vi "Open Message Handler.vi"(6 "Mouse Position":T1, 7 "User VI Ref":refnum<vi>, 8 "Is Multi-select?":bool, 9 "Remaining Items":refnum<vi>[](array[refnum]), 10 "Affected Items":cluster{"Refnums 1":refnum<vi>[]}, 11 "Menu Refnum":refnum<k9>) -> (3 "Menu Items To Add":T2[](array[typedef]))   [LabVIEW 2020]
doc: "This VI is part of a plug-in for modifying the LabVIEW shortcut menus. This is the builder VI which is called when the shortcut menu is built. It tells LabVIEW which shortcut menu items to add to the menu."
uses:
  <resource>/plugins/PopupMenus/support/Shortcut Menu Item Definition.ctl
  <resource>/plugins/PopupMenus/support/Transaction Control.ctl
  <resource>/plugins/PopupMenus/support/Position In Menu.ctl
  <resource>/plugins/PopupMenus/support/Relative Position.ctl
  <resource>/plugins/PopupMenus/support/Checkmark Status.ctl
  <resource>/plugins/PopupMenus/support/Enabled Menu Item Status.ctl
  <vilib>/Utility/miscctls.llb/LVPositionTypeDef.ctl
panel:
  # "Rules a popup plug-in must follow:\n* This VI's file name must match the file name of the LLB -- only the file extensions should be different.\n* This VI must have debugging disabled or it will be ignored as a plug-in.\n* For all menu items, \"tag suffix + file name of this VI\" must be less than 240 characters.\n* You can disconnect the \"Affected Items\" from the typedef to make the plug-in load faster. The typedef is only there to assist you in keeping this VI and the execution VI using to the same type.\n* All controls on this panel except \"Affected Items\" are locked to prevent accidental edits. Do not change the types or the names of controls other than the elements inside the \"Affected Items\" cluster.\n* See Context Help for more information on the individual controls."
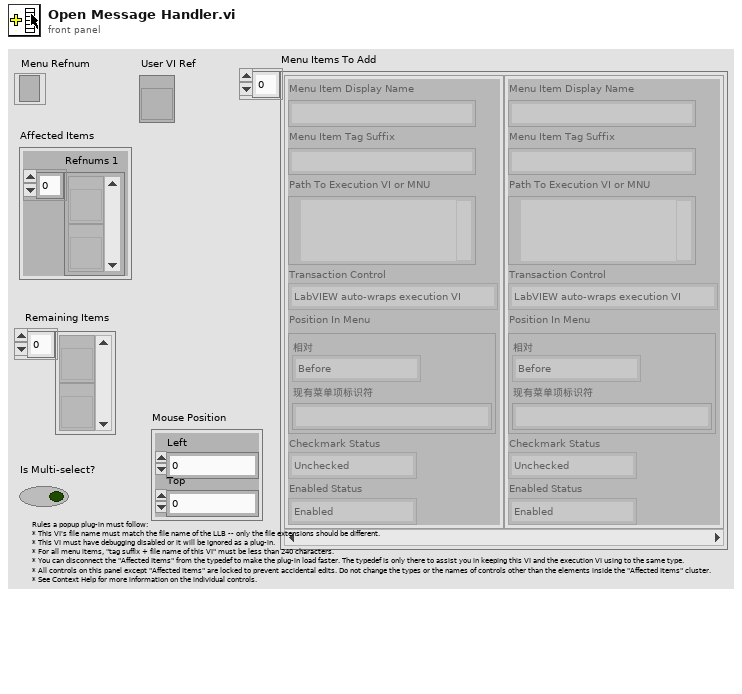
[diagram p1: front panel]
types:
  T1 = typedef "LVPositionTypeDef.ctl" = cluster{"Left":i32, "Top":i32}
  T2 = typedef "Shortcut Menu Item Definition.ctl" = cluster{"Menu Item Display Name":string, "Menu Item Tag Suffix":string, "Path To Execution VI or MNU":path, "Transaction Control":T3, "Position In Menu":T4, "Checkmark Status":T6, "Enabled Status":T7}
  T3 = typedef "Transaction Control.ctl" = enum8{"LabVIEW auto-wraps execution VI", "Execution VI will define if needed"}
  T4 = typedef "Position In Menu.ctl" = cluster{"Relative":T5, "Existing Item Tag":string}
  T5 = typedef "Relative Position.ctl" = enum8{"Before", "Instead of", "After", "Into Submenu"}
  T6 = typedef "Checkmark Status.ctl" = enum8{"Unchecked", "Checked"}
  T7 = typedef "Enabled Menu Item Status.ctl" = enum8{"Enabled", "Disabled"}
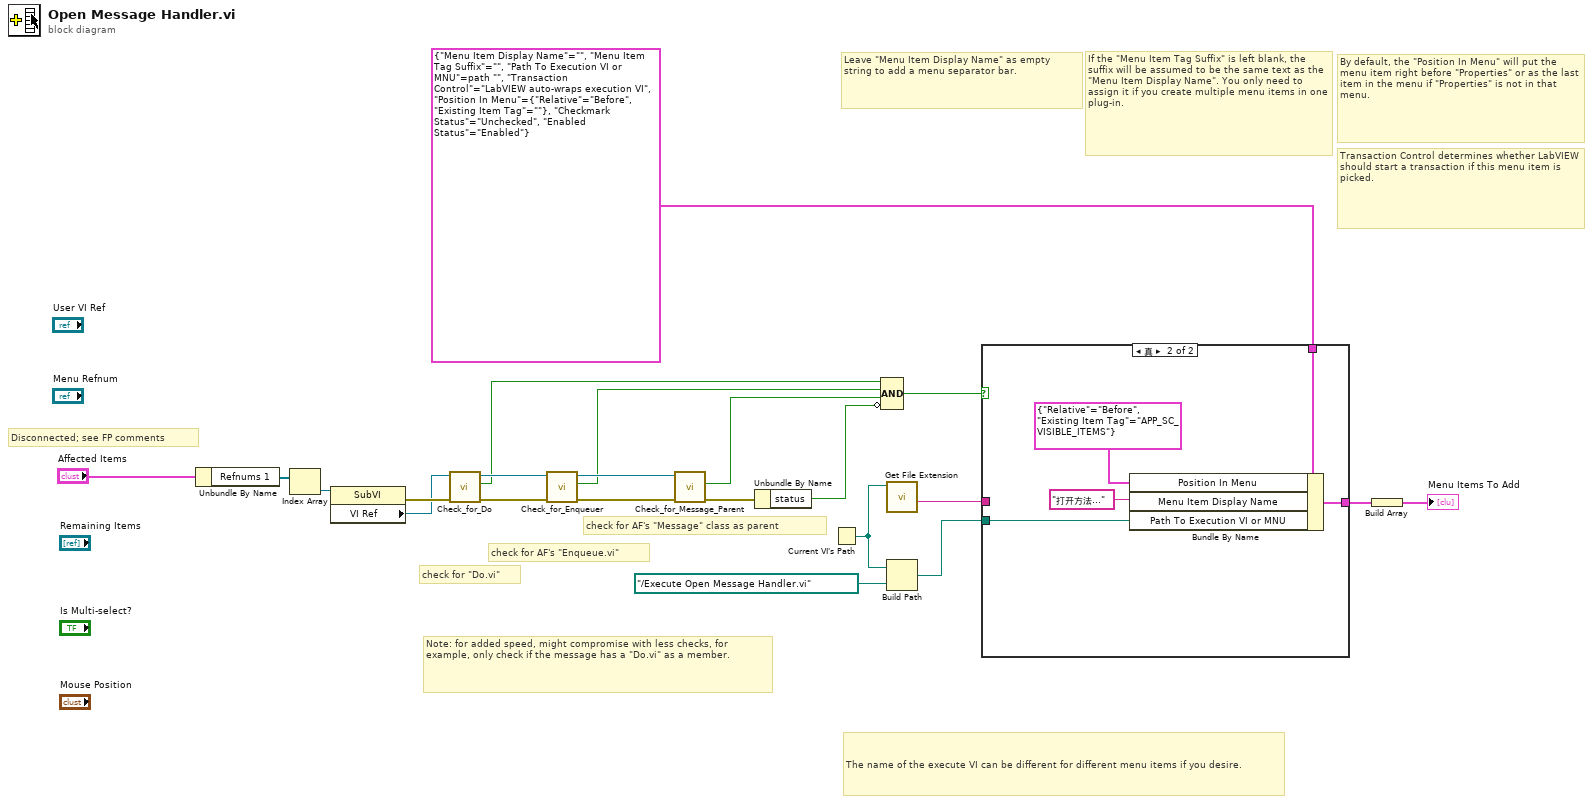
[diagram p0: block diagram]
diagram:
  # "Note: for added speed, might compromise with less checks, for example, only check if the message has a \"Do.vi\" as a member."
  # "check for AF's \"Message\" class as parent"
  # "check for AF's \"Enqueue.vi\""
  # "check for \"Do.vi\""
  # "Disconnected; see FP comments"
  # "Transaction Control determines whether LabVIEW should start a transaction if this menu item is picked."
  # "Leave \"Menu Item Display Name\" as empty string to add a menu separator bar."
  # "If the \"Menu Item Tag Suffix\" is left blank, the suffix will be assumed to be the same text as the \"Menu Item Display Name\". You only need to assign it if you create multiple menu items in one plug-in."
  # "By default, the \"Position In Menu\" will put the menu item right before \"Properties\" or as the last item in the menu if \"Properties\" is not in that menu."
  # "The name of the execute VI can be different for different menu items if you desire."
  n1 = Unbundle By Name("Affected Items") -> ("Refnums 1"=w13:refnum<vi>[])
  n2 = Index Array(array=w13) -> (element=w11:refnum<vi>)  [unwired: 1 in]
  n3 = property class="SubVI"(reference=w11) -> (error out=w22:errorcluster, "VI Ref"=w10:refnum<vi>)  [unwired: 1 in, 1 out]
  n4 = call "Check_for_Do.vi"("error in (no error)"=w22, "VI ref"=w10) -> ("error out"=w9:errorcluster, "Has Do.vi?"=w6:bool, "VI ref out"=w12:refnum<vi>)  [unwired: 6 in, 1 out]
  n5 = call "Check_for_Enqueuer.vi"("error in (no error)"=w9, "VI ref"=w12) -> ("error out"=w7:errorcluster, "Has Enqueuer?"=w5:bool, "VI ref out"=w8:refnum<vi>)  [unwired: 7 in]
  n6 = call "Check_for_Message_Parent.vi"("error in (no error)"=w7, "VI ref"=w8) -> ("error out"=w3:errorcluster, "Inherits from AF Message?"=w4:bool)  [unwired: 6 in, 2 out]
  n7 = Unbundle By Name(w3) -> ("status"=w1:bool)
  n8 = Current VI's Path() -> (path=w16:path)
  n9 = Compound Arithmetic op=AND(w6, w5, w4, invert w1) -> (w2:bool)
  n10 = call <vilib>:"Get File Extension.vi"("file"=w16) -> ("filename without extension"=w15:string)  [unwired: 6 in, 4 out]
  n11 = Build Path(base path=w16, name or relative path=path "../Execute Open Message Handler.vi" ("execute path")) -> (appended path=w20:path)
  n12 = case shown="真" w2 {
    tunnel: w20 -> [_ w27]
    tunnel: T2 {"Menu Item Display Name"="", "Menu Item Tag Suffix"="", "Path To Execution VI or MNU"=path "", "Transaction Control"=enum."LabVIEW auto-wraps execution VI", "Position In Menu"={"Relative"=enum."Before", "Existing Item Tag"=""}, "Checkmark Status"=enum."Unchecked", "Enabled Status"=enum."Enabled"} ("Cluster") -> [_ w26]
    tunnel: [_ w25] -> w18
    tunnel: w15 -> [_ _]
    frame False {
    }
    frame True {
      n13 = Bundle By Name(cluster=w26, "Position In Menu"=T4 {"Relative"=enum."Before", "Existing Item Tag"="APP_SC_VISIBLE_ITEMS"}, "Menu Item Display Name"="打开方法...", "Path To Execution VI or MNU"=w27) -> (w25:T2)
    }
  }
  n14 = Build Array(w18) -> (→"Menu Items To Add":T2[])
